vi "Command Type.vi"(11 "HTTP Command Config in":refnum<class "HTTP Command Config.lvclass">) -> (2 "Command Type":T1)   [LabVIEW 2020, in "VolatusSeqConfig.lvlib" / "HTTP Command Config.lvclass"]
uses:
  HTTP Command Config.lvclass
  HTTP Command Config.lvclass/HTTP Command Config.ctl
  Command Type.ctl
  VolatusSeqConfig.lvlib
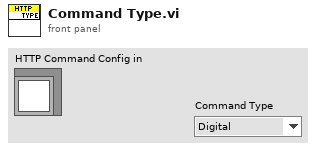
[diagram p1: front panel]
types:
  T1 = typedef "VolatusSeqConfig.lvlib/Command Type.ctl" = enum16{"Digital", "Numeric", "Transition", "Stop", "StartLog", "StopLog", "Start", "Event", "Error", "HTTP"}
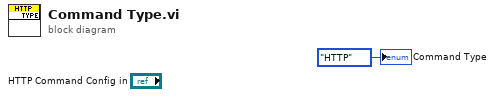
[diagram p0: block diagram]
diagram:
  "Command Type" <- Command_Type."HTTP" ("Command Type")
